vi "Pfeiffer TPG361-mul-reads-average.vi"(8 "error in (no error)":errorcluster, 10 "# reads to average":i32=1, 11 "VISA Refnum in":refnum<visa-resource-name>) -> (0 "error out":errorcluster, 1 "Pressure CH1":dbl, 2 "Status Sensor 1":i32(ring) items=["data OK", "underrange", "overrange", "sensor error", "sensor off", "no sensor", "ID error"], 3 "VISA Refnum out":refnum<visa-resource-name>)   [LabVIEW 2019]
uses:
  <vilib>/Analysis/baseanly.llb/Mean (DBL).vi
  <instrlib>/PV ActiveLine/Public/Data/PV ActiveLine - Measurement Data all Gauges (TPG362).vi
  <instrlib>/PV ActiveLine/PV ActiveLine.lvlib
  <vilib>/Analysis/NI_AALBase.lvlib
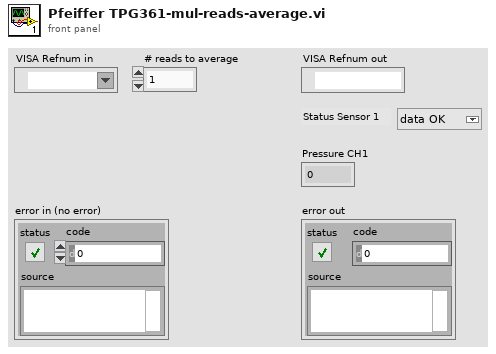
[diagram p1: front panel]
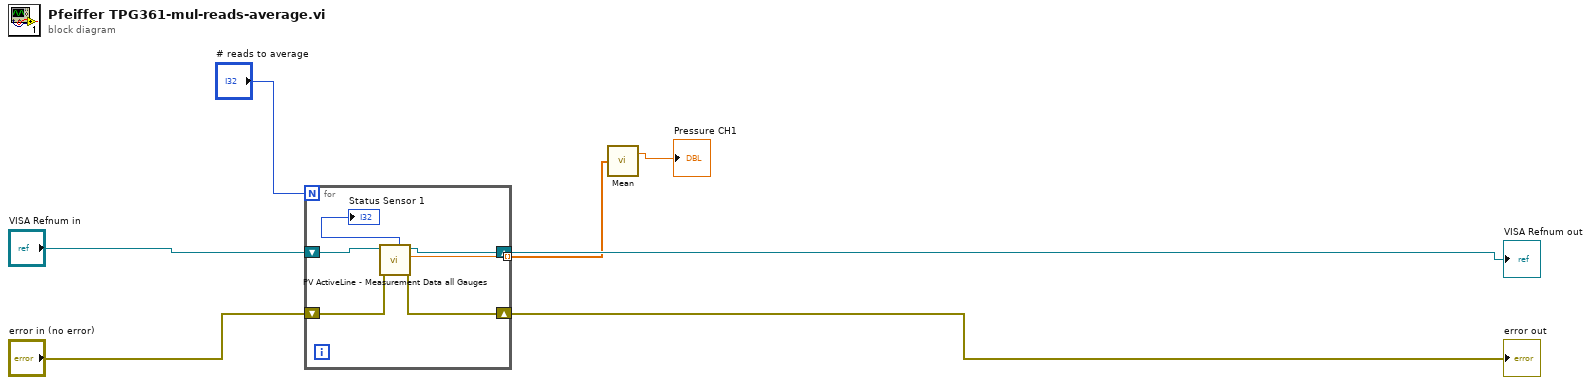
[diagram p0: block diagram]
diagram:
  n1 = for {
    N: "# reads to average" -> [_]
    tunnel: [w9] -> w2 mode=indexing
    shift-right: [w12] -> w5
    shift-left: "VISA Refnum in" -> [w13]
    shift-right: [w11] -> w6
    shift-left: "error in (no error)" -> [w8]
    n2 = call-poly <instrlib>:"PV ActiveLine - Measurement Data all Gauges.vi"("Fehler (Eingang)"=w8, "Referenz in"=w13) -> ("Cluster (Ausgang)"=w11:errorcluster, "Pressure CH1"=w9:dbl, "Referenz out"=w12:refnum<visa-resource-name>, "Status CH1"=→"Status Sensor 1":i32)  [unwired: 4 in, 2 out]
  }
  "error out" <- w6
  "VISA Refnum out" <- w5
  n3 = call-poly <vilib>:"Mean.vi"("X"=w2) -> ("mean"=→"Pressure CH1":dbl)  [unwired: 1 out]
